vi "fgv_DCAF INI Refnum.vi"(10 "Action":T1, 11 "INI Refnum In":T2) -> (3 "INI Refnum Out":T2)   [LabVIEW 2014, in "Standard Editor.lvlib" / "DCAF INI.lvlib"]
doc: "FGV to store DCAF INI reference."
uses:
  DCAF INI.lvlib
  <vilib>/Utility/config.llb/Config Data RefNum.ctl
  enum_DCAF INI FGV Action.ctl
  <vilib>/Utility/config.llb/NI_LVConfig.lvlib
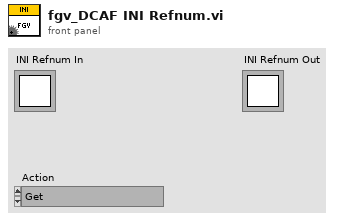
[diagram p1: front panel]
types:
  T1 = typedef "Standard Editor.lvlib/DCAF INI.lvlib/enum_DCAF INI FGV Action.ctl" = enum16{"Get", "Set"}
  T2 = typedef "NI_LVConfig.lvlib/Config Data RefNum.ctl" = refnum<k1>
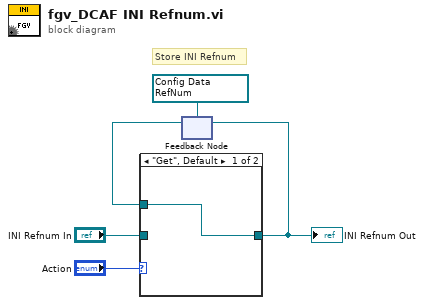
[diagram p0: block diagram]
diagram:
  w1 = T2 refnum items=["config data"] ("refnum")
  # "Store INI Refnum"
  n1 = feedback #1(w1) -> (w2:T2)
  n2 = case shown="\"Get\", Default" "Action" {
    tunnel: "INI Refnum In" -> [_ w7]
    tunnel: [w6 w7] -> w3
    tunnel: w2 -> [w6 _]
    frame "Get", Default {
    }
    frame "Set" {
    }
  }
  "INI Refnum Out" <- w3
  n3 = feedback-in #1(w3) -> ()
